vi "MKS670_Global.vi"() -> ()   [LabVIEW 2019]
panel:
  out "MKS670_He3_P":dbl
  out "MKS670_He3_ST":u32(colorbox)
  out "MKS670_100_ST":u32(colorbox)
  out "MKS670_100_P":dbl
  out "MKS670_1000_ST":u32(colorbox)
  out "MKS670_1000_P":dbl
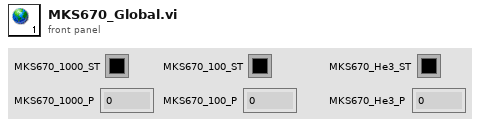
[diagram p1: front panel]
diagram:
